vi "Simulated Temperature.vi"(1 "Temperature Units":enum32{"Celsius", "Farenheit"}(radio)=enum."Farenheit") -> (0 "Thermometer":dbl(slide) scale=0.0..100.0)   [LabVIEW 2011]
doc: "This VI simulates acquiring temperature data one value at a time from a plug-in data acquisition board. You can also select whether the temperature is displayed in degrees Fahrenheit or degrees Celsius."
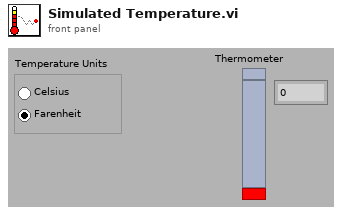
[diagram p1: front panel]
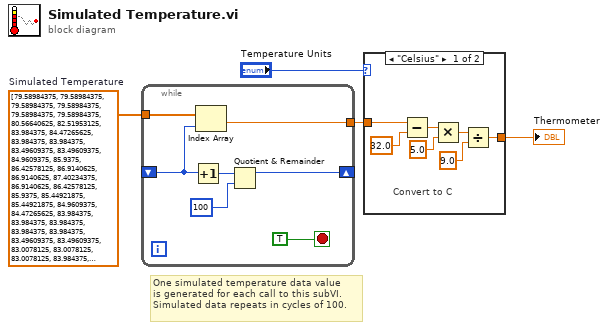
[diagram p0: block diagram]
diagram:
  w2 = dbl[] [79.58984375, 79.58984375, 79.58984375, 79.58984375, 79.58984375, 79.58984375, 80.56640625, 82.51953125, 83.984375, 84.47265625, 83.984375, 83.984375, 83.49609375, 83.49609375, 84.9609375, 85.9375, 86.42578125, 86.9140625, 86.9140625, 87.40234375, 86.9140625, 86.42578125, 85.9375, 85.44921875, 85.44921875, 84.9609375, 84.47265625, 83.984375, 83.984375, 83.984375, 83.984375, 83.984375, 83.49609375, 83.49609375, 83.0078125, 83.0078125, 83.0078125, 83.984375, 84.47265625, 84.9609375, 85.44921875, 86.42578125, 86.9140625, 86.9140625, 86.9140625, 86.42578125, 85.9375, 85.44921875, 85.9375, 86.9140625, 87.40234375, 87.890625, 87.40234375, 86.9140625, 86.9140625, 85.9375, 85.9375, 85.9375, 84.9609375, 84.9609375, 84.9609375, 84.47265625, 84.47265625, 85.44921875, 85.9375, 86.9140625, 86.9140625, 86.42578125, 85.9375, 85.44921875, 85.44921875, 84.9609375, 84.9609375, 84.47265625, 84.47265625, 83.984375, 83.984375, 83.49609375, 83.49609375, 83.0078125, 83.0078125, 83.0078125, 83.0078125, 83.0078125, 83.0078125, 83.0078125, 82.51953125, 81.0546875, 81.54296875, 82.51953125, 83.0078125, 82.51953125, 82.03125, 82.03125, 82.03125, 82.03125, 81.54296875, 81.54296875, 81.54296875, 81.54296875]  # Simulated Temperature
  # "One simulated temperature data value \nis generated for each call to this subVI.  \nSimulated data repeats in cycles of 100."
  n1 = while {
    tunnel: w2 -> [w6]
    tunnel: [w7] -> w1
    shift-left: _ -> [w11]
    shift-right: [w8] -> _
    stop <- TRUE stop-if-true
    n2 = Increment(x=w11) -> (x+1=w10:i32)
    n3 = Index Array(array=w6, index=w11) -> (element=w7:dbl)
    n4 = Quotient & Remainder(x=w10, y=100) -> (x-y*floor(x/y)=w8:i32)  [unwired: 1 out]
  }
  n5 = case shown="\"Celsius\"" "Temperature Units" {
    tunnel: [w13 w19] -> w3
    tunnel: w1 -> [w12 w19]
    frame "Celsius" {
      # "Convert to C"
      n6 = Subtract(x=w12, y=32.0) -> (x-y=w18:dbl)
      n7 = Multiply(x=w18, y=5.0) -> (x*y=w17:dbl)
      n8 = Divide(x=w17, y=9.0) -> (x/y=w13:dbl)
    }
    frame "Farenheit", Default {
    }
  }
  "Thermometer" <- w3
